vi "F22.vi"(8 "error in (no error)":errorcluster, 9 "data":u8[](array[numeric]), 10 "function":u8, 11 "device data model in":refnum<class "Standard Data Model.lvclass">) -> (0 "error out":errorcluster, 1 "data return":u8[](array[numeric]), 2 "function return":u8, 3 "device data model out":refnum<class "Standard Data Model.lvclass">)   [LabVIEW 2017, in "SubVIs.lvlib" / "Standard Data Model.lvclass"]
doc: "Executes function code 22"
uses:
  <vilib>/Modbus/subvis/Data and Functions/Standard Data Model/Standard Data Model.lvclass
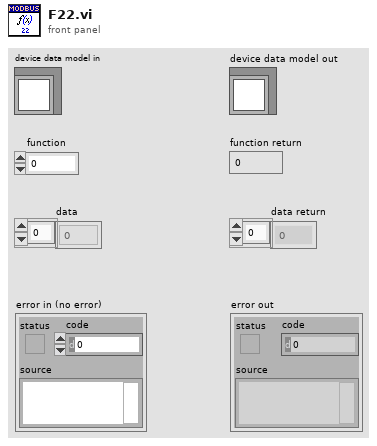
[diagram p1: front panel]
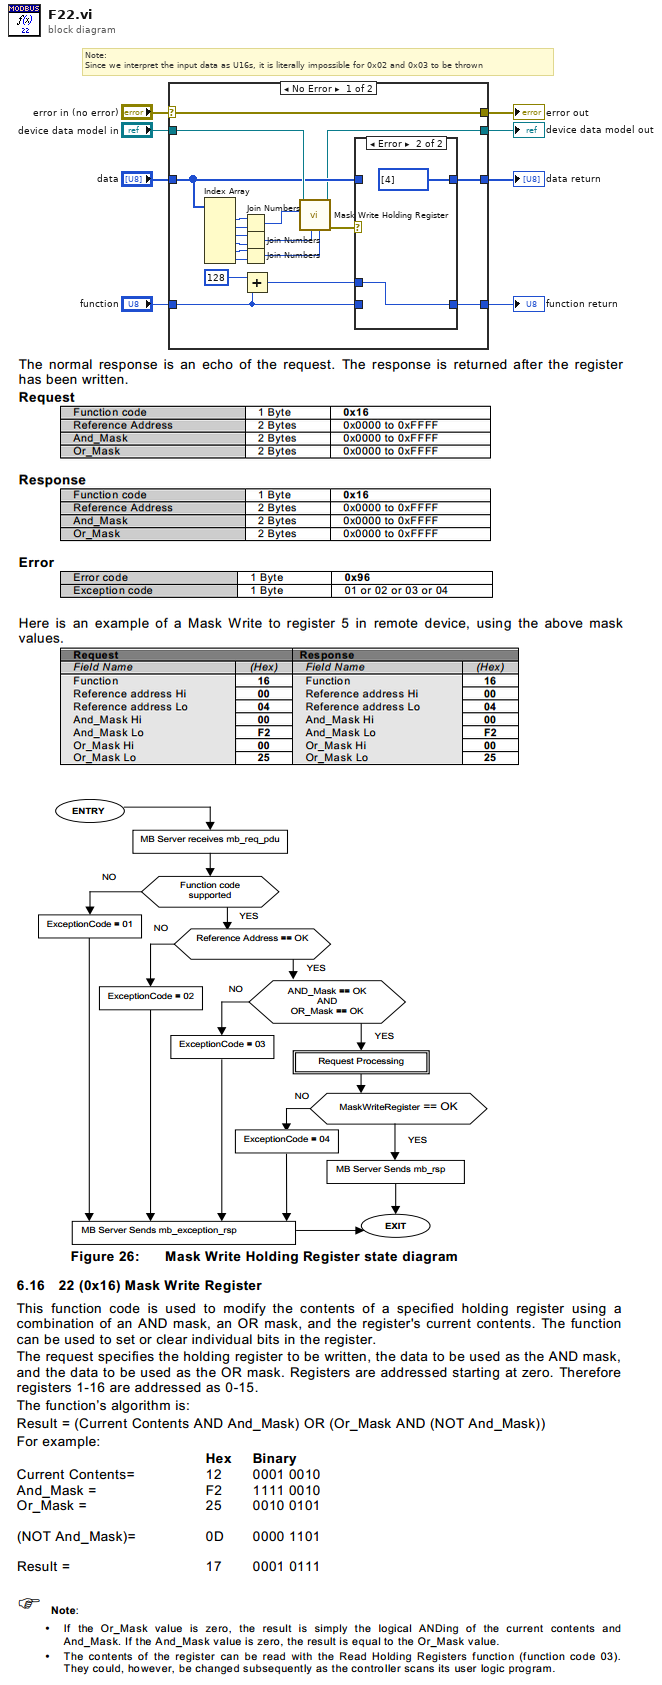
[diagram p0: block diagram]
diagram:
  # "Note:\nSince we interpret the input data as U16s, it is literally impossible for 0x02 and 0x03 to be thrown"
  n1 = case shown="No Error" "error in (no error)" {
    selector: "error in (no error)" -> [w27 w35]
    tunnel: [w27 w35] -> w7
    tunnel: [w9 w34] -> w5
    tunnel: "device data model in" -> [w15 w34]
    tunnel: "function" -> [w20 w33]
    tunnel: "data" -> [w10 w32]
    tunnel: [w19 w33] -> w2
    tunnel: [w18 w32] -> w1
    frame No Error {
      n2 = Index Array(array=w10) -> (element #1=w25:u8, element #2=w26:u8, element #3=w24:u8, element #4=w23:u8, element #5=w16:u8, element #6=w17:u8)  [unwired: 6 in]
      n3 = Join Numbers(hi=w25, lo=w26) -> ((hi.lo)=w14:u16)
      n4 = Join Numbers(hi=w24, lo=w23) -> ((hi.lo)=w13:u16)
      n5 = Join Numbers(hi=w16, lo=w17) -> ((hi.lo)=w12:u16)
      n6 = Add(x=u8 128, y=w20) -> (x+y=w21:u8)
      n7 = call-dynamic "Mask Write Holding Register.vi"("OR mask"=w12, "AND mask"=w13, "address"=w14, "device data model in"=w15) -> ("error out"=w11:errorcluster, "device data model out"=w9:refnum<class "Standard Data Model.lvclass">)  [unwired: 6 in]
      n8 = case shown="Error" w11 {
        tunnel: w21 -> [_ w31]
        tunnel: w20 -> [w29 _]
        tunnel: [w29 w31] -> w19
        tunnel: [w28 u8[] [4]] -> w18
        tunnel: w10 -> [w28 _]
        frame No Error {
        }
        frame Error {
        }
      }
    }
    frame Error {
    }
  }
  "error out" <- w7
  "device data model out" <- w5
  "data return" <- w1
  "function return" <- w2
